vi "Лабораторная №1 Задание 3_7.vi"() -> ()   [LabVIEW 2017]
panel:
  out "Текущее время":string
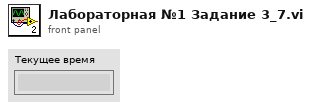
[diagram p1: front panel]
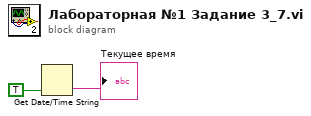
[diagram p0: block diagram]
diagram:
  n1 = Get Date/Time String(want seconds? (F)=TRUE) -> (time string=→"Текущее время":string)  [unwired: 2 in, 1 out]
